vi "ACQ control.vi"(0 "events fets propi Refnum":refnum<vi>, 1 "events fets altre Refnum":refnum<vi>, 2 "Total events Refnum":refnum<vi>, 5 "ACQ stop by events":T1={"ACQ stop by events button"=FALSE, "Events to acquire"=1000} caption="Stop by events" {"Events to acquire" min=1}, 6 "events per comm":u32, 7 "Stop ACQ button Refnum":refnum<vi>, 8 "comm error or timeout":bool, 9 "Acquisition time Refnum":refnum<vi>, 11 "Actual time Refnum":refnum<vi>, 12 "events propi":u32, 13 "start time (in seconds)":dbl, 15 "ACQ barra Refnum":refnum<vi>, 16 "STOP FPGAs Refnum":refnum<vi>) -> (21 "Stop by events":bool)   [LabVIEW 2015, in "VIPM2.lvlib"]
doc: "FGV to sum events. FGV to stop FPGAs."
uses:
  VIPM2.lvlib
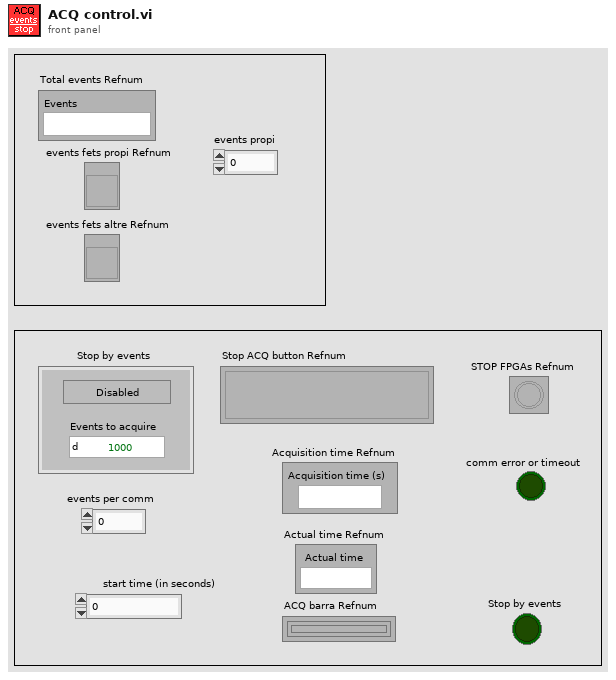
[diagram p1: front panel]
types:
  T1 = cluster{"ACQ stop by events button":bool, "Events to acquire":u32}
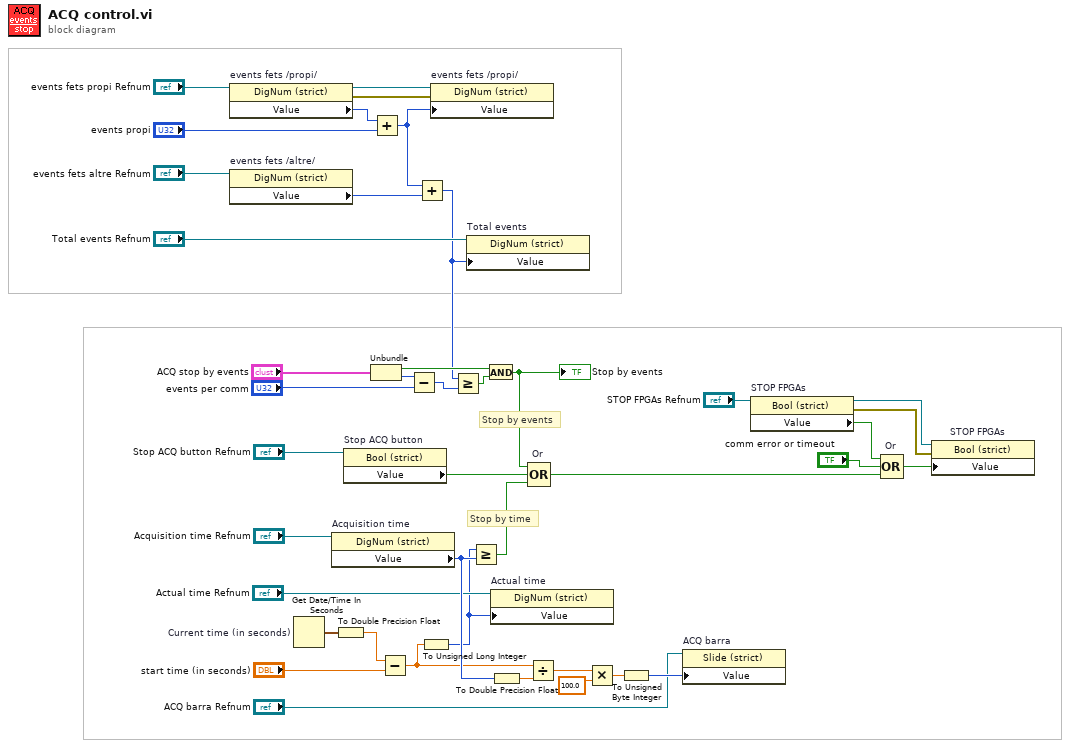
[diagram p0: block diagram]
diagram:
  # "Stop by events"
  # "Stop by time"
  n1 = property on="events fets /propi/" class="DigNum (strict)"(reference="events fets propi Refnum") -> (reference out=w41:refnum<vi>, error out=w40:errorcluster, "Value"=w37:u32)  [unwired: 1 in]
  n2 = property on="events fets /altre/" class="DigNum (strict)"(reference="events fets altre Refnum") -> ("Value"=w38:u32)  [unwired: 1 in, 2 out]
  n3 = Get Date/Time In Seconds "Current time (in seconds)"() -> (seconds since 1Jan1904=w4:timestamp)
  n4 = property on="Acquisition time" class="DigNum (strict)"(reference="Acquisition time Refnum") -> ("Value"=w23:u32)  [unwired: 1 in, 2 out]
  n5 = To Double Precision Float(number=w4) -> (double precision float=w3:dbl)
  n6 = property on="Stop ACQ button" class="Bool (strict)"(reference="Stop ACQ button Refnum") -> ("Value"=w21:bool)  [unwired: 1 in, 2 out]
  n7 = Unbundle("ACQ stop by events") -> ("ACQ stop by events button"=w31:bool, "Events to acquire"=w29:u32)
  n8 = Add(x=w37, y="events propi") -> (x+y=w39:u32)
  n9 = Subtract(x=w3, y="start time (in seconds)") -> (x-y=w1:dbl)
  n10 = Subtract(x=w29, y="events per comm") -> (x-y=w28:u32)
  n11 = Add(x=w39, y=w38) -> (x+y=w18:u32)
  n12 = To Unsigned Long Integer(number=w1) -> (unsigned 32bit integer=w2:u32)
  n13 = property on="events fets /propi/" class="DigNum (strict)"(reference=w41, error in=w40, "Value"=w39) -> ()  [unwired: 2 out]
  n14 = Greater Or Equal?(x=w18, y=w28) -> (x >= y?=w30:bool)
  n15 = property on="Total events" class="DigNum (strict)"(reference="Total events Refnum", "Value"=w18) -> ()  [unwired: 1 in, 2 out]
  n16 = Greater Or Equal?(x=w2, y=w23) -> (x >= y?=w32:bool)
  n17 = And(x=w31, y=w30) -> (x .and. y?=w12:bool)
  "Stop by events" <- w12
  n18 = property on="Actual time" class="DigNum (strict)"(reference="Actual time Refnum", "Value"=w2) -> ()  [unwired: 1 in, 2 out]
  n19 = To Double Precision Float(number=w23) -> (double precision float=w24:dbl)
  n20 = Compound Arithmetic op=OR "Or"(w12, w21, w32) -> (w11:bool)
  n21 = Divide(x=w1, y=w24) -> (x/y=w25:dbl)
  n22 = Multiply(x=w25, y=100.0) -> (x*y=w27:dbl)
  n23 = To Unsigned Byte Integer(number=w27) -> (unsigned 8bit integer=w22:u8)
  n24 = property on="ACQ barra" class="Slide (strict)"(reference="ACQ barra Refnum", "Value"=w22) -> ()  [unwired: 1 in, 2 out]
  n25 = property on="STOP FPGAs" class="Bool (strict)"(reference="STOP FPGAs Refnum") -> (reference out=w6:refnum<vi>, error out=w5:errorcluster, "Value"=w8:bool)  [unwired: 1 in]
  n26 = Compound Arithmetic op=OR "Or"(w8, "comm error or timeout", w11) -> (w7:bool)
  n27 = property on="STOP FPGAs" class="Bool (strict)"(reference=w6, error in=w5, "Value"=w7) -> ()  [unwired: 2 out]
